vi "Waypoint Transfer Status.vi"   [LabVIEW 2014]
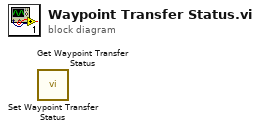
[diagram p0: block diagram]
diagram:
  n1 = call "Set Waypoint Transfer Status.vi"() -> ()  [unwired: 11 in, 1 out]
  n2 = call "Get Waypoint Transfer Status.vi"() -> ()  [unwired: 10 in, 2 out]
